vi "RC_test_reader.vi"(8 "error in (no error)":errorcluster, 9 "Motors IDs Found":u8[](array[numeric]), 10 "Read positions (dyn)":dbl[](array[numeric]), 11 "VISA Refnum in":refnum<visa-resource-name>) -> (0 "error out":errorcluster[](array[cluster]), 2 "Dynamixel Positions (deg)":dbl[](array[numeric]), 3 "Read positions latest (dyn)":dbl[](array[numeric]))   [LabVIEW 2013]
doc: "This VI takes an array of motor IDs and reads the position of each one. It outputs as both raw values and as degrees.\n\nIt's set up for the SAIL Dynamixels, because it scales by 360/1200. We're still investigating whether the rudder has different units."
uses:
  <instrlib>/Dynamixel Motor/Dynamixel Motor.lvlib
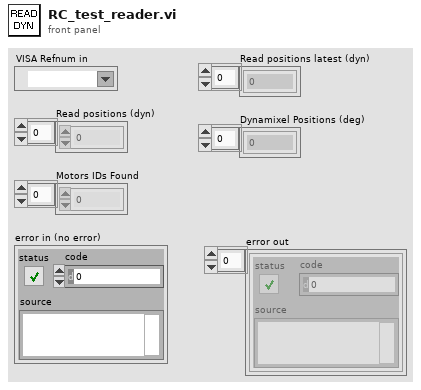
[diagram p1: front panel]
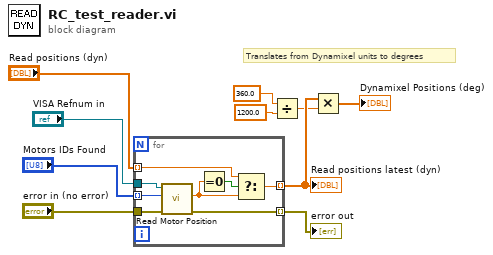
[diagram p0: block diagram]
diagram:
  # "Translates from Dynamixel units to degrees"
  n1 = for {
    tunnel: "VISA Refnum in" -> [w18]
    tunnel: [w12] -> w9 mode=indexing
    tunnel: "Motors IDs Found" -> [w15] mode=indexing
    tunnel: "error in (no error)" -> [w17]
    tunnel: [w16] -> w4 mode=indexing
    tunnel: "Read positions (dyn)" -> [w11] mode=indexing
    n2 = call <instrlib>:"Read Motor Position.vi"("error in (no error)"=w17, "Motor ID (0)"=w15, "VISA resource name"=w18) -> ("error out"=w16:errorcluster, "Position (deg)"=w13:dbl)  [unwired: 6 in, 1 out]
    n3 = Equal To 0?(x=w13) -> (x = 0?=w14:bool)
    n4 = Select(t=w11, s=w14, f=w13) -> (s? t:f=w12:dbl)
  }
  "Read positions latest (dyn)" <- w9
  "error out" <- w4
  n5 = Divide(x=360.0, y=1200.0) -> (x/y=w8:dbl)
  n6 = Multiply(x=w9, y=w8) -> (x*y=→"Dynamixel Positions (deg)":dbl[])
